vi "[RT]Loop_Controller.vi"(8 "error in (no error)":errorcluster, 11 "Queue in":refnum<queue>) -> (0 "error out":errorcluster)   [LabVIEW 2018]
uses:
  TypeDef/CMD Cluster.ctl
  TypeDef/ControllerState.ctl
  [GlobVar]SensorState.vi
panel:
  in  "myRIO BefehlsQueue":refnum<queue>
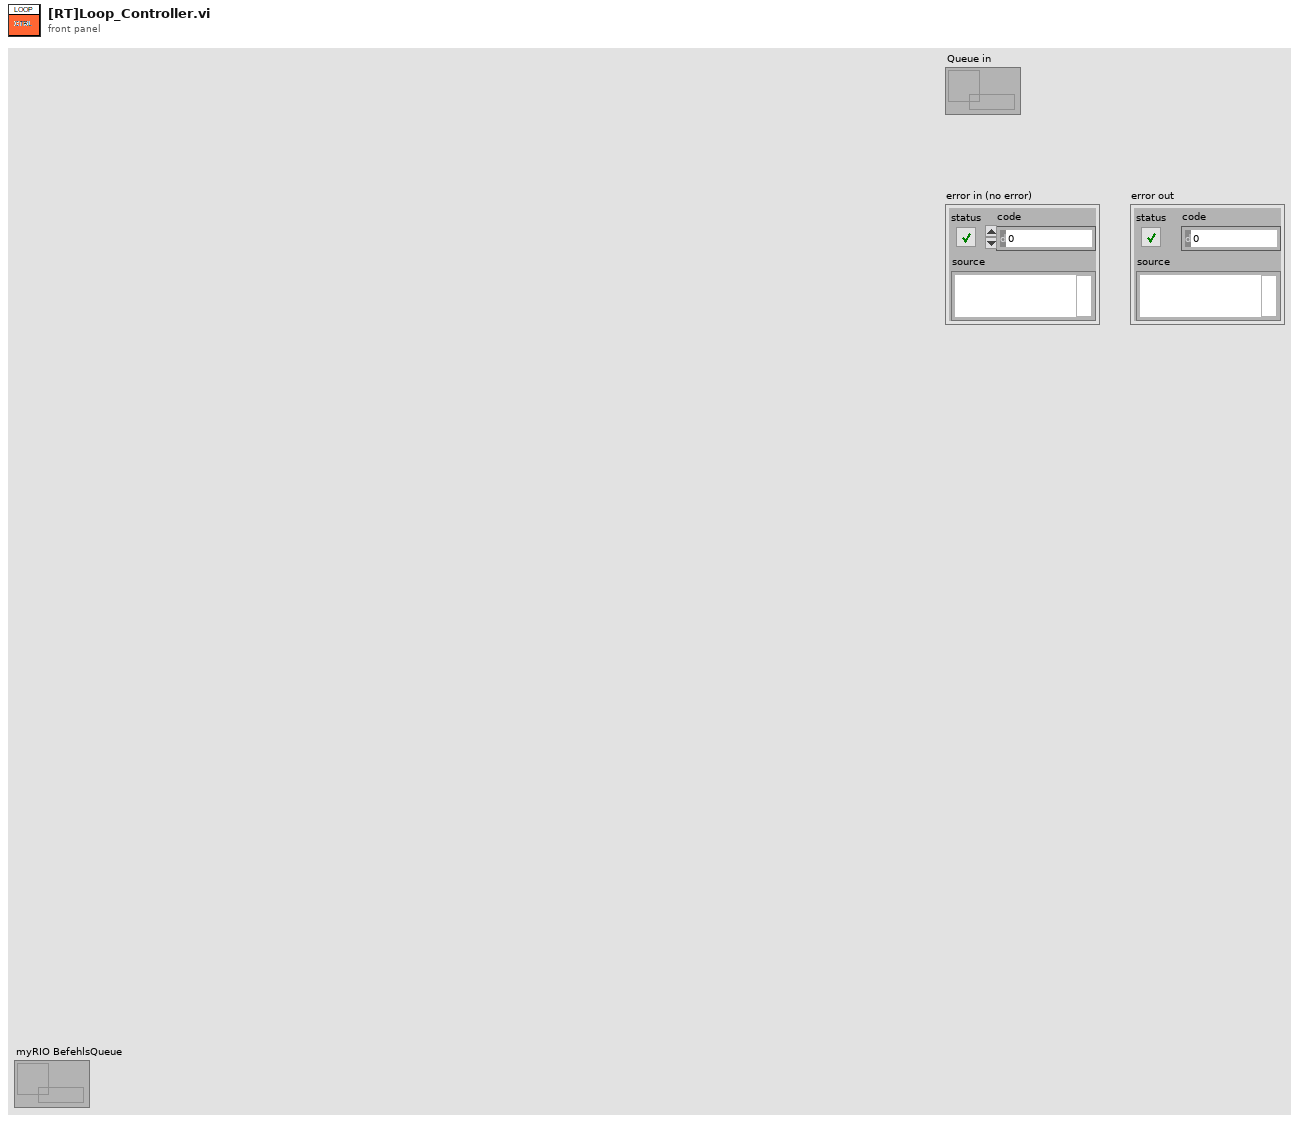
[diagram p1: front panel]
types:
  T1 = typedef "ControllerState.ctl" = enum16{"Idle", "Vorheizen", "Brühen", "Emergency-Stop"}
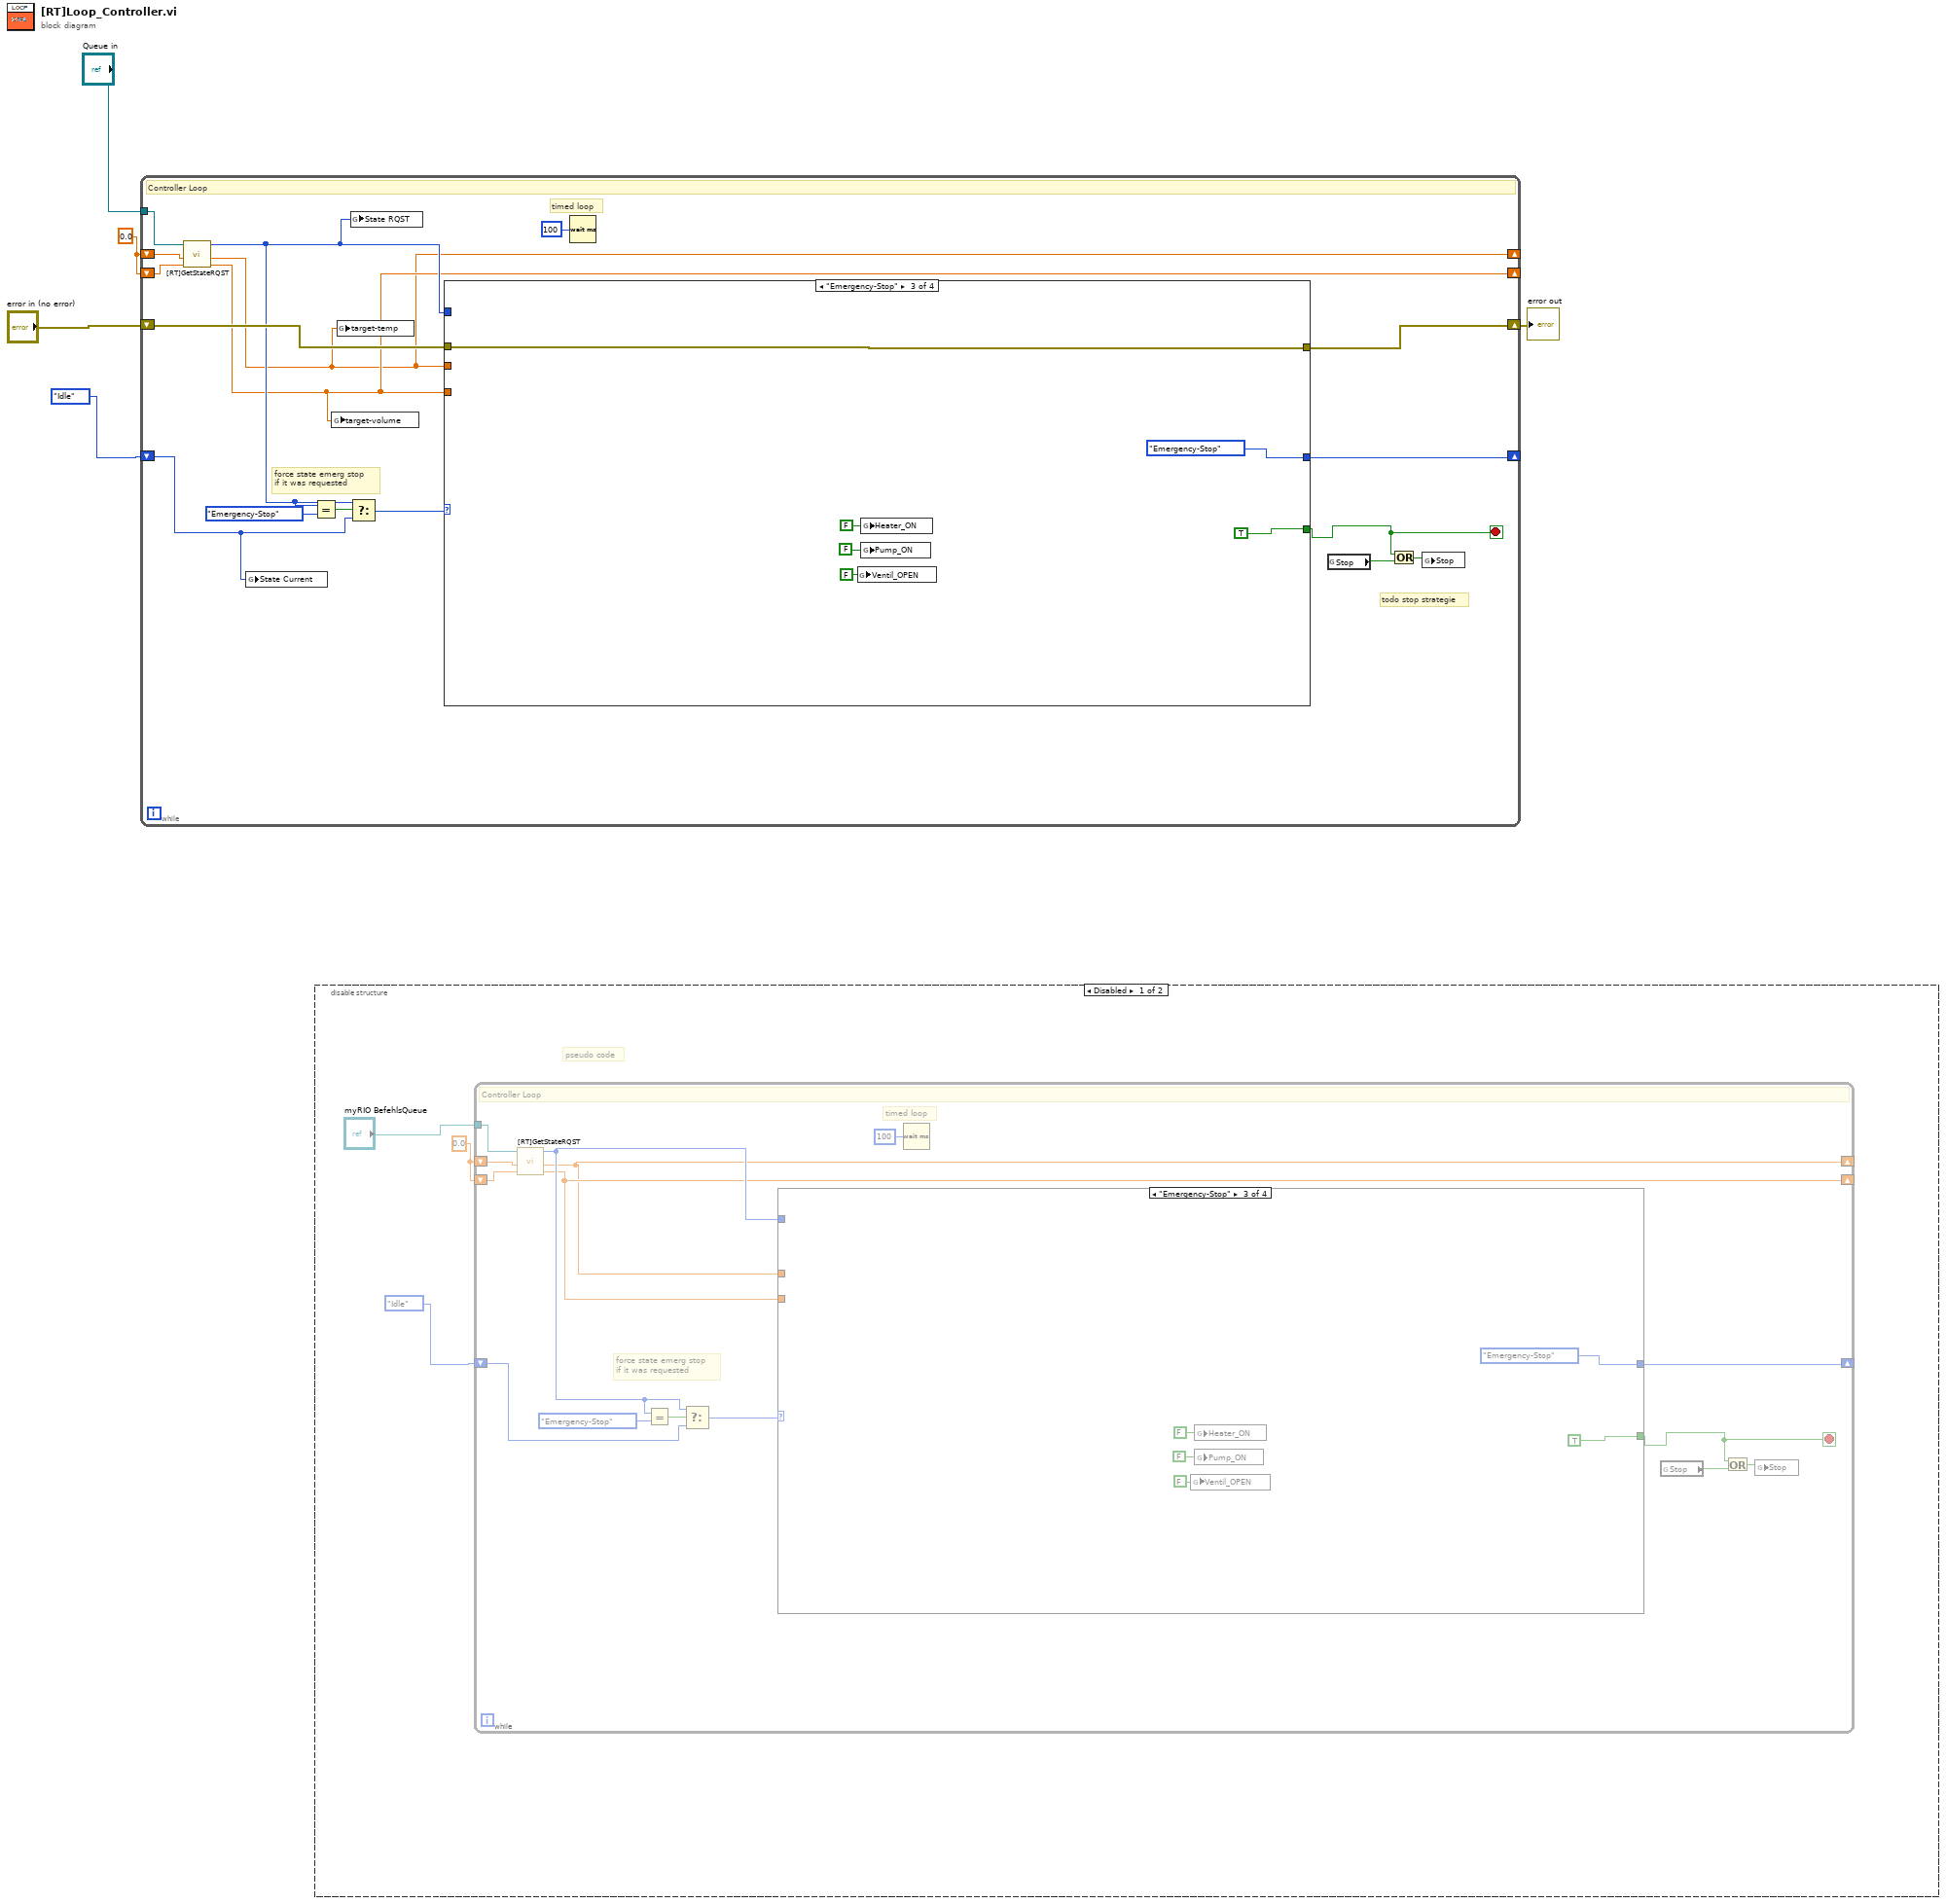
[diagram p0: block diagram]
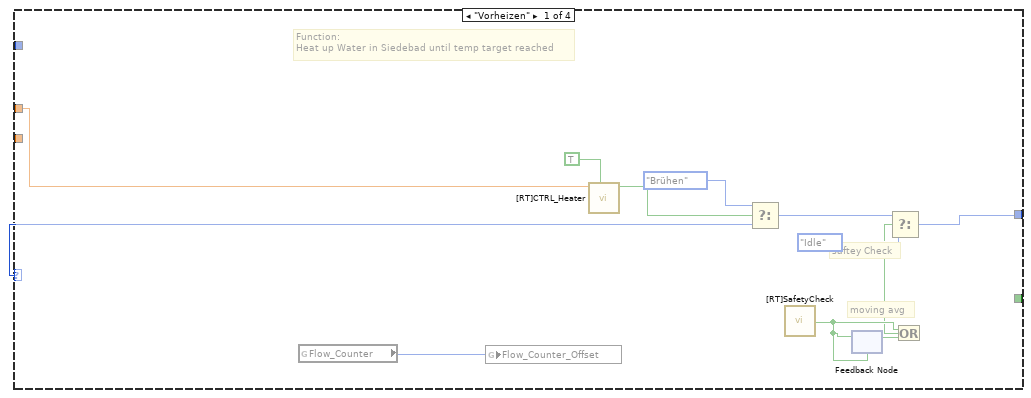
[diagram p2: hidden frame]
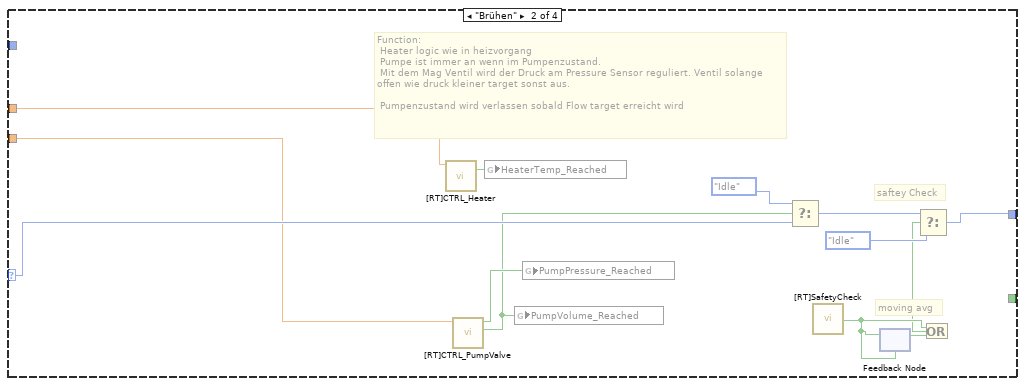
[diagram p3: hidden frame]
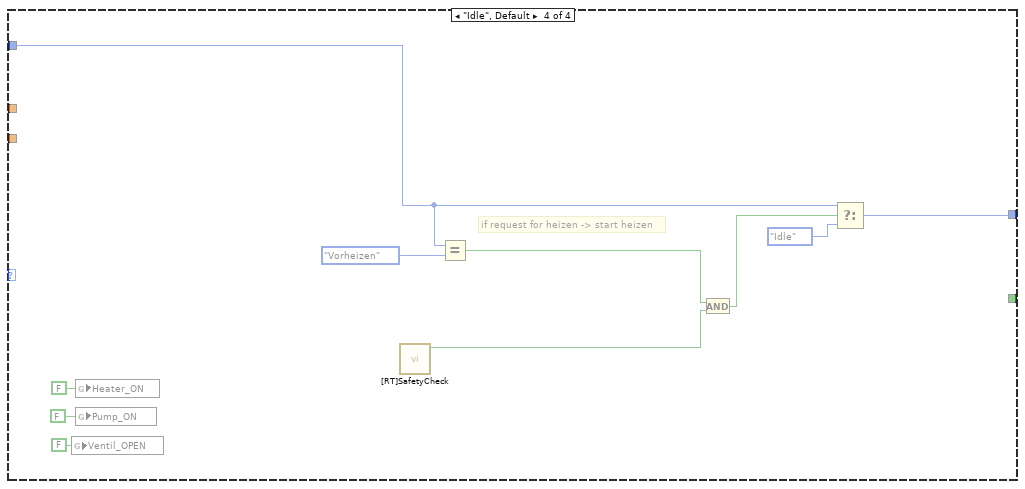
[diagram p4: hidden frame]
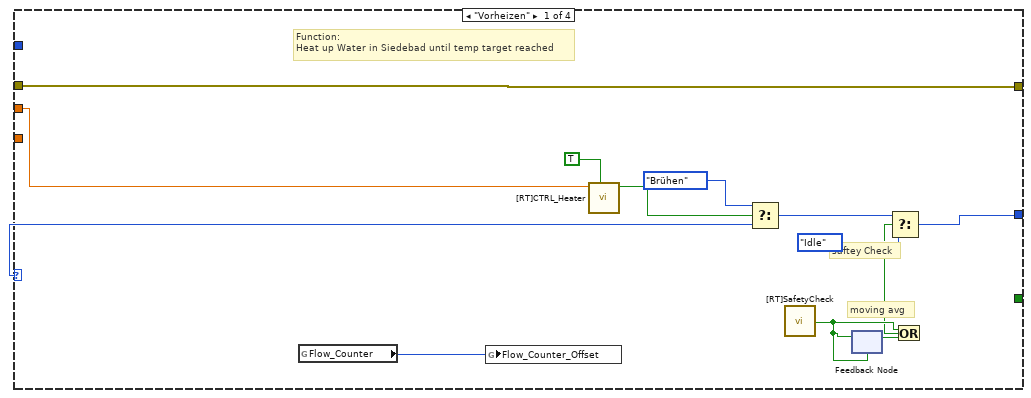
[diagram p6: hidden frame]
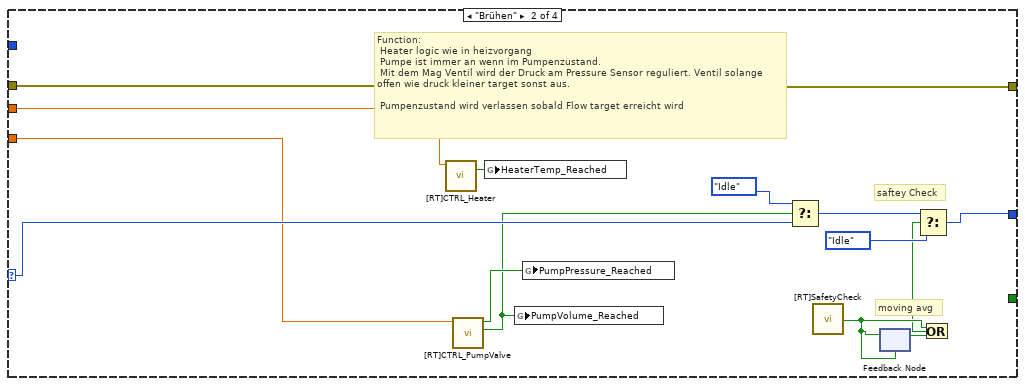
[diagram p7: hidden frame]
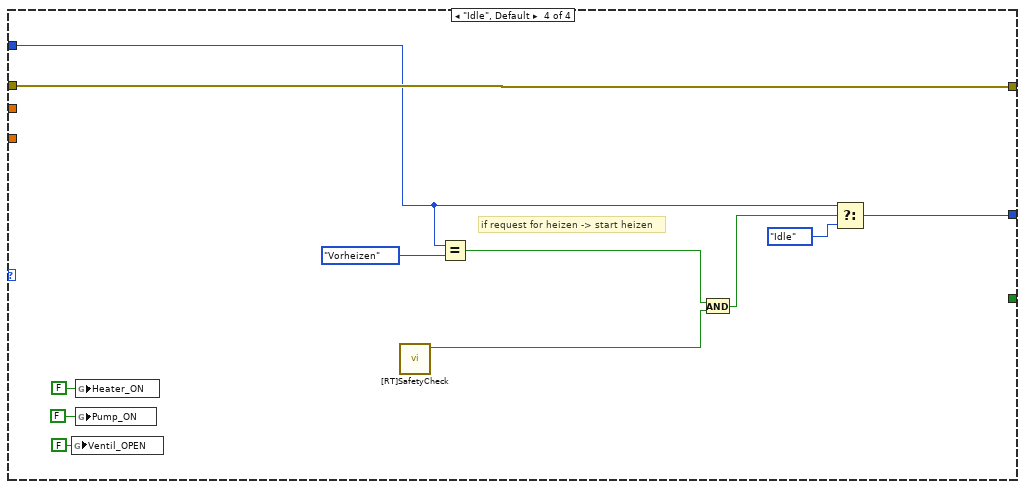
[diagram p8: hidden frame]
diagram:
  w5 = 0.0 ("target-volume")
  n1 = while {
    shift-right: [w21] -> w3
    shift-left: "error in (no error)" -> [w22]
    shift-right: [w20] -> _
    shift-left: ControllerState."Idle" -> [w9]
    tunnel: "Queue in" -> [w19]
    shift-right: [w7] -> _
    shift-left: w5 -> [w10]
    shift-right: [w6] -> _
    shift-left: w5 -> [w11]
    stop <- w12 stop-if-true
    # "todo stop strategie"
    # "force state emerg stop \nif it was requested"
    # "timed loop"
    # "Controller Loop"
    n2 = call "[RT]GetStateRQST.vi"("target-volume out"=w10, "target-temp in"=w11, "Queue in"=w19) -> ("target-volume"=w7:dbl, "target-temp"=w6:dbl, "State Rqst"=w8:T1)  [unwired: 6 in]
    n3 = global write "[GlobVar]SensorState.vi" "State Current"(w9) -> ()
    n4 = Equal?(x=w8, y=ControllerState."Emergency-Stop") -> (x = y?=w17:bool)
    n5 = global write "[GlobVar]SensorState.vi" "target-volume"(w7) -> ()
    n6 = global write "[GlobVar]SensorState.vi" "target-temp"(w6) -> ()
    n7 = global write "[GlobVar]SensorState.vi" "State RQST"(w8) -> ()
    n8 = Select(t=w8, s=w17, f=w9) -> (s? t:f=w15:T1)
    n9 = case shown="\"Emergency-Stop\"" w15 {
      selector: w15 -> [w34 w47 _ _]
      tunnel: w22 -> [w35 w49 w55 w66]
      tunnel: [w35 w49 w55 w66] -> w21
      tunnel: [_ _ TRUE _] -> w12
      tunnel: [w23 w39 ControllerState."Emergency-Stop" w65] -> w20
      tunnel: w8 -> [_ _ _ w62]
      tunnel: w6 -> [w32 w46 _ _]
      tunnel: w7 -> [_ w42 _ _]
      frame "Vorheizen" {
        # "saftey Check"
        # "moving avg"
        # "Function: \nHeat up Water in Siedebad until temp target reached"
        n10 = global read "[GlobVar]SensorState.vi" "Flow_Counter"() -> (w30:u64)
        n11 = global write "[GlobVar]SensorState.vi" "Flow_Counter_Offset"(w30) -> ()
        n12 = call "[RT]CTRL_Heater.vi"("vorheizen?"=TRUE, "target-temp"=w32) -> ("temp_reached"=w31:bool)  [unwired: 9 in]
        n13 = Select(t=ControllerState."Brühen", s=w31, f=w34) -> (s? t:f=w24:T1)
        n14 = call "[RT]SafetyCheck.vi"() -> ("No_Error"=w26:bool)  [unwired: 11 in]
        n15 = feedback #1(w26) -> (w27:bool)
        n16 = feedback-in #1(w26) -> ()
        n17 = Or(x=w26, y=w27) -> (x .or. y?=w25:bool)
        n18 = Select(t=w24, s=w25, f=ControllerState."Idle") -> (s? t:f=w23:T1)
      }
      frame "Brühen" {
        # "saftey Check"
        # "moving avg"
        # "Function:\n\tHeater logic wie in heizvorgang\n\tPumpe ist immer an wenn im Pumpenzustand.\n\tMit dem Mag Ventil wird der Druck am Pressure Sensor reguliert. Ventil solange offen wie druck kleiner target sonst aus.\n\t\n\tPumpenzustand wird verlassen sobald Flow target erreicht wird"
        n19 = call "[RT]CTRL_Heater.vi"("target-temp"=w46) -> ("temp_reached"=w45:bool)  [unwired: 10 in]
        n20 = call "[RT]CTRL_PumpValve.vi"("target-volume"=w42) -> ("volume reached"=w43:bool, "pressure reached"=w44:bool)  [unwired: 9 in]
        n21 = global write "[GlobVar]SensorState.vi" "HeaterTemp_Reached"(w45) -> ()
        n22 = global write "[GlobVar]SensorState.vi" "PumpVolume_Reached"(w43) -> ()
        n23 = global write "[GlobVar]SensorState.vi" "PumpPressure_Reached"(w44) -> ()
        n24 = Select(t=ControllerState."Idle", s=w43, f=w47) -> (s? t:f=w40:T1)
        n25 = call "[RT]SafetyCheck.vi"() -> ("No_Error"=w37:bool)  [unwired: 11 in]
        n26 = feedback #2(w37) -> (w38:bool)
        n27 = feedback-in #2(w37) -> ()
        n28 = Or(x=w37, y=w38) -> (x .or. y?=w36:bool)
        n29 = Select(t=w40, s=w36, f=ControllerState."Idle") -> (s? t:f=w39:T1)
      }
      frame "Emergency-Stop" {
        n30 = global write "[GlobVar]SensorState.vi" "Ventil_OPEN"(FALSE ("Heater_ON")) -> ()
        n31 = global write "[GlobVar]SensorState.vi" "Heater_ON"(FALSE ("Heater_ON")) -> ()
        n32 = global write "[GlobVar]SensorState.vi" "Pump_ON"(FALSE ("Heater_ON")) -> ()
      }
      frame "Idle", Default {
        # "if request for heizen -> start heizen"
        n33 = global write "[GlobVar]SensorState.vi" "Ventil_OPEN"(FALSE ("Heater_ON")) -> ()
        n34 = global write "[GlobVar]SensorState.vi" "Heater_ON"(FALSE ("Heater_ON")) -> ()
        n35 = global write "[GlobVar]SensorState.vi" "Pump_ON"(FALSE ("Heater_ON")) -> ()
        n36 = call "[RT]SafetyCheck.vi"() -> ("No_Error"=w58:bool)  [unwired: 11 in]
        n37 = Equal?(x=w62, y=ControllerState."Vorheizen") -> (x = y?=w57:bool)
        n38 = And(x=w57, y=w58) -> (x .and. y?=w56:bool)
        n39 = Select(t=w62, s=w56, f=ControllerState."Idle") -> (s? t:f=w65:T1)
      }
    }
    n40 = Wait (ms)(milliseconds to wait=u32 100) -> ()  [unwired: 1 out]
    n41 = global read "[GlobVar]SensorState.vi" "Stop"() -> (w14:bool)
    n42 = Or(x=w12, y=w14) -> (x .or. y?=w13:bool)
    n43 = global write "[GlobVar]SensorState.vi" "Stop"(w13) -> ()
  }
  "error out" <- w3
  n44 = disable-structure shown="Disabled" {
    frame Disabled {
      w69 = 0.0 ("target-volume")
      # "pseudo code"
      n45 = while {
        shift-right: [w84] -> _
        shift-left: ControllerState."Idle" -> [w73]
        tunnel: "myRIO BefehlsQueue" -> [w83]
        shift-right: [w71] -> _
        shift-left: w69 -> [w74]
        shift-right: [w70] -> _
        shift-left: w69 -> [w75]
        stop <- w76 stop-if-true
        # "force state emerg stop \nif it was requested"
        # "timed loop"
        # "Controller Loop"
        n46 = call "[RT]GetStateRQST.vi"("target-volume out"=w74, "target-temp in"=w75, "Queue in"=w83) -> ("target-volume"=w71:dbl, "target-temp"=w70:dbl, "State Rqst"=w72:T1)  [unwired: 6 in]
        n47 = Equal?(x=w72, y=ControllerState."Emergency-Stop") -> (x = y?=w81:bool)
        n48 = Select(t=w72, s=w81, f=w73) -> (s? t:f=w79:T1)
        n49 = case shown="\"Emergency-Stop\"" w79 {
          selector: w79 -> [w96 w108 _ _]
          tunnel: [_ _ TRUE _] -> w76
          tunnel: [w85 w100 ControllerState."Emergency-Stop" w124] -> w84
          tunnel: w72 -> [_ _ _ w121]
          tunnel: w70 -> [w94 w107 _ _]
          tunnel: w71 -> [_ w103 _ _]
          frame "Vorheizen" {
            # "saftey Check"
            # "moving avg"
            # "Function: \nHeat up Water in Siedebad until temp target reached"
            n50 = global read "[GlobVar]SensorState.vi" "Flow_Counter"() -> (w92:u64)
            n51 = global write "[GlobVar]SensorState.vi" "Flow_Counter_Offset"(w92) -> ()
            n52 = call "[RT]CTRL_Heater.vi"("vorheizen?"=TRUE, "target-temp"=w94) -> ("temp_reached"=w93:bool)  [unwired: 9 in]
            n53 = Select(t=ControllerState."Brühen", s=w93, f=w96) -> (s? t:f=w86:T1)
            n54 = call "[RT]SafetyCheck.vi"() -> ("No_Error"=w88:bool)  [unwired: 11 in]
            n55 = feedback #3(w88) -> (w89:bool)
            n56 = feedback-in #3(w88) -> ()
            n57 = Or(x=w88, y=w89) -> (x .or. y?=w87:bool)
            n58 = Select(t=w86, s=w87, f=ControllerState."Idle") -> (s? t:f=w85:T1)
          }
          frame "Brühen" {
            # "saftey Check"
            # "moving avg"
            # "Function:\n\tHeater logic wie in heizvorgang\n\tPumpe ist immer an wenn im Pumpenzustand.\n\tMit dem Mag Ventil wird der Druck am Pressure Sensor reguliert. Ventil solange offen wie druck kleiner target sonst aus.\n\t\n\tPumpenzustand wird verlassen sobald Flow target erreicht wird"
            n59 = call "[RT]CTRL_Heater.vi"("target-temp"=w107) -> ("temp_reached"=w106:bool)  [unwired: 10 in]
            n60 = call "[RT]CTRL_PumpValve.vi"("target-volume"=w103) -> ("volume reached"=w104:bool, "pressure reached"=w105:bool)  [unwired: 9 in]
            n61 = global write "[GlobVar]SensorState.vi" "HeaterTemp_Reached"(w106) -> ()
            n62 = global write "[GlobVar]SensorState.vi" "PumpVolume_Reached"(w104) -> ()
            n63 = global write "[GlobVar]SensorState.vi" "PumpPressure_Reached"(w105) -> ()
            n64 = Select(t=ControllerState."Idle", s=w104, f=w108) -> (s? t:f=w101:T1)
            n65 = call "[RT]SafetyCheck.vi"() -> ("No_Error"=w98:bool)  [unwired: 11 in]
            n66 = feedback #4(w98) -> (w99:bool)
            n67 = feedback-in #4(w98) -> ()
            n68 = Or(x=w98, y=w99) -> (x .or. y?=w97:bool)
            n69 = Select(t=w101, s=w97, f=ControllerState."Idle") -> (s? t:f=w100:T1)
          }
          frame "Emergency-Stop" {
            n70 = global write "[GlobVar]SensorState.vi" "Ventil_OPEN"(FALSE ("Heater_ON")) -> ()
            n71 = global write "[GlobVar]SensorState.vi" "Heater_ON"(FALSE ("Heater_ON")) -> ()
            n72 = global write "[GlobVar]SensorState.vi" "Pump_ON"(FALSE ("Heater_ON")) -> ()
          }
          frame "Idle", Default {
            # "if request for heizen -> start heizen"
            n73 = global write "[GlobVar]SensorState.vi" "Ventil_OPEN"(FALSE ("Heater_ON")) -> ()
            n74 = global write "[GlobVar]SensorState.vi" "Heater_ON"(FALSE ("Heater_ON")) -> ()
            n75 = global write "[GlobVar]SensorState.vi" "Pump_ON"(FALSE ("Heater_ON")) -> ()
            n76 = call "[RT]SafetyCheck.vi"() -> ("No_Error"=w117:bool)  [unwired: 11 in]
            n77 = Equal?(x=w121, y=ControllerState."Vorheizen") -> (x = y?=w116:bool)
            n78 = And(x=w116, y=w117) -> (x .and. y?=w115:bool)
            n79 = Select(t=w121, s=w115, f=ControllerState."Idle") -> (s? t:f=w124:T1)
          }
        }
        n80 = Wait (ms)(milliseconds to wait=u32 100) -> ()  [unwired: 1 out]
        n81 = global read "[GlobVar]SensorState.vi" "Stop"() -> (w78:bool)
        n82 = Or(x=w76, y=w78) -> (x .or. y?=w77:bool)
        n83 = global write "[GlobVar]SensorState.vi" "Stop"(w77) -> ()
      }
    }
    frame Enabled {
    }
  }
